vi "QueueMotorStart.vi"(1 "MotorNum":refnum<queue>, 2 "Step":refnum<queue>, 3 "Direction":refnum<queue>, 5 "错误输入（无错误）":errorcluster, 6 "MotorNum_Int":i32, 8 "Step_Int":i32, 10 "Direction_Int":i32) -> (15 "MotorNum_OUT":refnum<queue>, 16 "Step_OUT":refnum<queue>, 17 "Direction_OUT":refnum<queue>, 19 "错误输出":errorcluster)   [LabVIEW 2011]
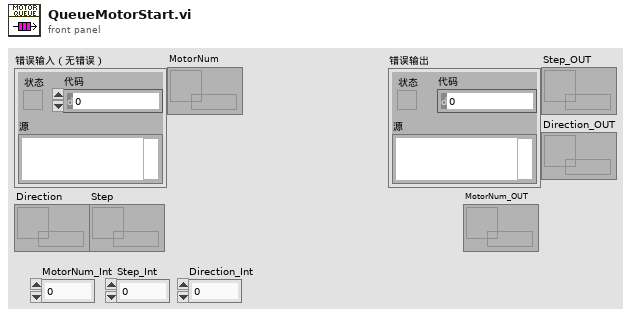
[diagram p1: front panel]
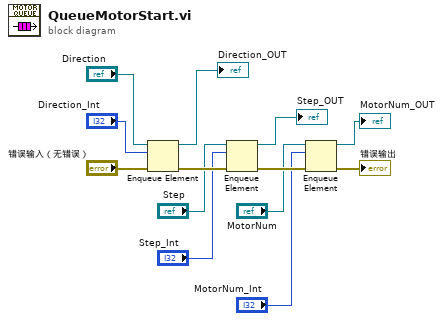
[diagram p0: block diagram]
diagram:
  n1 = Enqueue Element(queue="Direction", element="Direction_Int", error in (no error)="错误输入（无错误）") -> (queue out=→"Direction_OUT":refnum<queue>, error out=w13:errorcluster)  [unwired: 1 in, 1 out]
  n2 = Enqueue Element(queue="Step", element="Step_Int", error in (no error)=w13) -> (queue out=→"Step_OUT":refnum<queue>, error out=w12:errorcluster)  [unwired: 1 in, 1 out]
  n3 = Enqueue Element(queue="MotorNum", element="MotorNum_Int", error in (no error)=w12) -> (queue out=→"MotorNum_OUT":refnum<queue>, error out=→"错误输出":errorcluster)  [unwired: 1 in, 1 out]
